vi "Actor Template_Launch-Static Link.vi"(5 "My Data":bool, 9 "Timeout":i32=1000 format="%dmsec", 11 "error in":errorcluster) -> (4 "FTW Actor Connector":refnum<class "FTW-ActorConnector.lvclass">, 6 "Initialized Response":string, 8 "Instance Inbox Address":string, 15 "error out":errorcluster)   [LabVIEW 2013]
uses:
  source/actor/Connector/FTW-ActorConnector.lvclass
  Core/Actor Template-Core_Process.vi
  Core/Actor Template-Core.lvclass
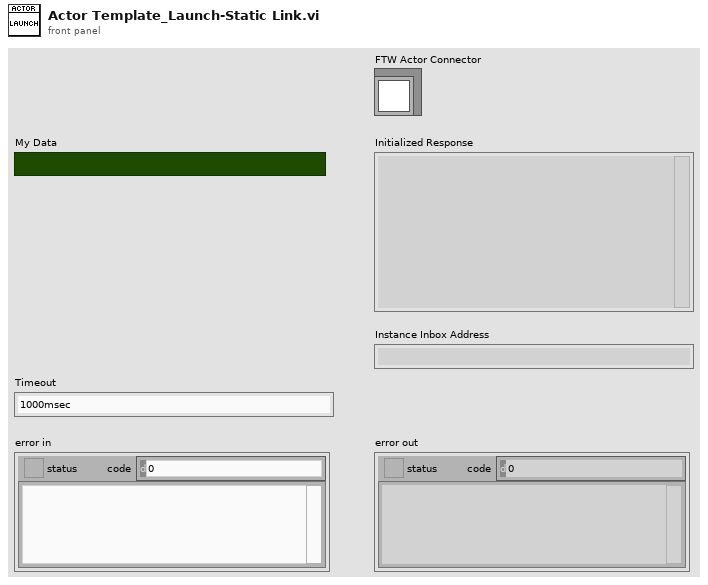
[diagram p1: front panel]
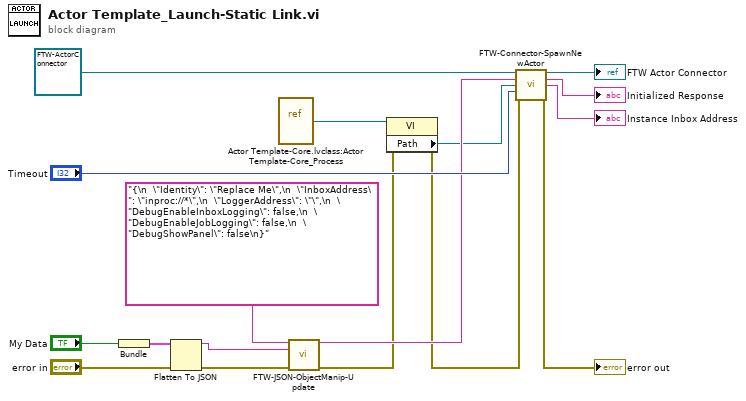
[diagram p0: block diagram]
diagram:
  n1 = Bundle("My Data"="My Data") -> (w8:cluster{"My Data":bool})  [unwired: 1 in]
  n2 = Flatten To JSON(anything=w8, error in (no error)="error in") -> (JSON string=w5:string, 11:w7:errorcluster)  [unwired: 1 in]
  n3 = vi-ref "Actor Template-Core.lvclass:Actor Template-Core_Process.vi"() -> (w9:refnum<vi>)
  n4 = call "FTW-JSON-ObjectManip-Update.vi"("Input JSON Object"="{\n  \"Identity\": \"Replace Me\",\n  \"InboxAddress\": \"inproc://*\",\n  \"LoggerAddress\": \"\",\n  \"DebugEnableInboxLogging\": false,\n  \"DebugEnableJobLogging\": false,\n  \"DebugShowPanel\": false\n}" ("Configuration"), "JSON Object to Merge"=w5, "error in"=w7) -> ("Output JSON Object"=w4:string, "error out"=w2:errorcluster)  [unwired: 11 in]
  n5 = property class="VI"(reference=w9, error in=w2) -> (error out=w1:errorcluster, "Path"=w3:path)  [unwired: 1 out]
  n6 = call "FTW-Connector-SpawnNewActor.vi"("FTW Actor Connector Type"=refnum<class "FTW-ActorConnector.lvclass"> refnum ("TTK_Splashscreen.lvclass"), "Configuration"=w4, "Actor VI Filepath"=w3, "Timeout"="Timeout", "error in"=w1) -> ("FTW Actor Connector"=→"FTW Actor Connector":refnum<class "FTW-ActorConnector.lvclass">, "Initialized Response"=→"Initialized Response":string, "Instance Inbox Address"=→"Instance Inbox Address":string, "error out"=→"error out":errorcluster)  [unwired: 7 in]
